vi "Send Command.vi"(8 "error in (no error)":errorcluster, 10 "Data cluster in":T1, 11 "VISA Refnum in":refnum<visa-resource-name>) -> (0 "error out":errorcluster, 2 "Data cluster out":T1, 3 "VISA Refnum out":refnum<visa-resource-name>)   [LabVIEW 2020]
uses:
  Data Cluster.ctl
panel:
  # "Send Data:"
  # "Receive Data:"
  # "Send Data:"
  # "Receive Data:"
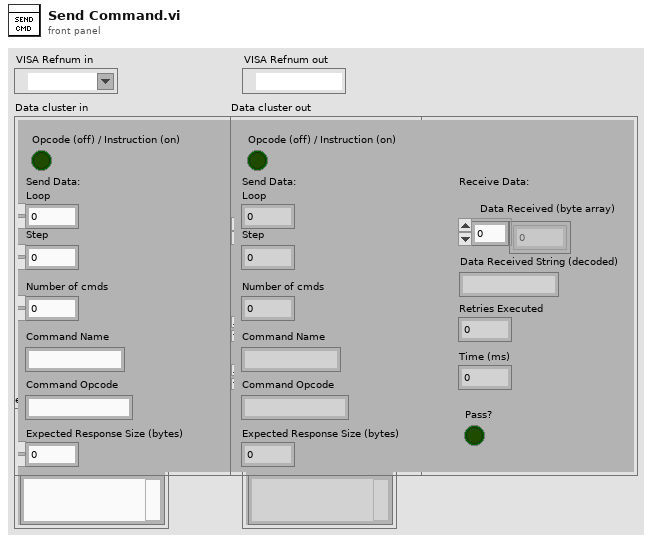
[diagram p1: front panel]
types:
  T1 = typedef "Data Cluster.ctl" = cluster{"Command Name":string, "Command Opcode ":string, "Step":dbl, "Loop":dbl, "Expected Response Size (bytes)":u16, "Number of cmds":dbl, "Data Received (byte array)":u8[], "Retries Executed":u16, "Time (ms)":u16, "Pass?":bool, "Opcode (off) / Instruction (on)":bool, "Data Received String (decoded)":string}
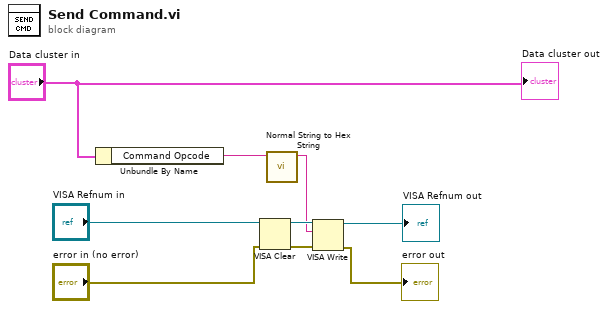
[diagram p0: block diagram]
diagram:
  n1 = Unbundle By Name("Data cluster in") -> ("Command Opcode"=w1:string)
  n2 = VISA Clear(VISA resource name="VISA Refnum in", error in (no error)="error in (no error)") -> (VISA resource name out=w4:refnum<visa-resource-name>, error out=w7:errorcluster)
  n3 = call "Normal String to Hex String.vi"("Command Opcode"=w1) -> ("Hex String"=w2:string)  [unwired: 10 in]
  n4 = VISA Write(VISA resource name=w4, write buffer=w2, error in (no error)=w7) -> (VISA resource name out=→"VISA Refnum out":refnum<visa-resource-name>, error out=→"error out":errorcluster)  [unwired: 1 out]
  "Data cluster out" <- "Data cluster in"
